vi "HelpOn.vi"(8 "Error In":errorcluster, 11 "object in":refnum<class "HelpInterface.lvclass">) -> (0 "Error Out":errorcluster, 3 "object out":refnum<class "HelpInterface.lvclass">)   [LabVIEW 2020, in "HelpInterface.lvclass"]
uses:
  HelpInterface.lvclass
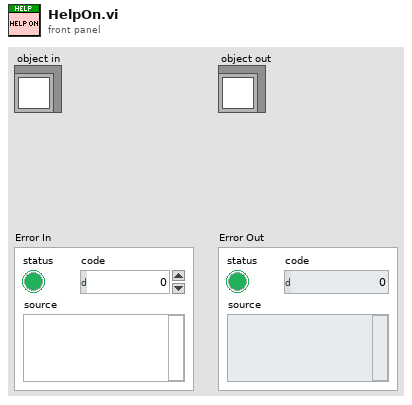
[diagram p1: front panel]
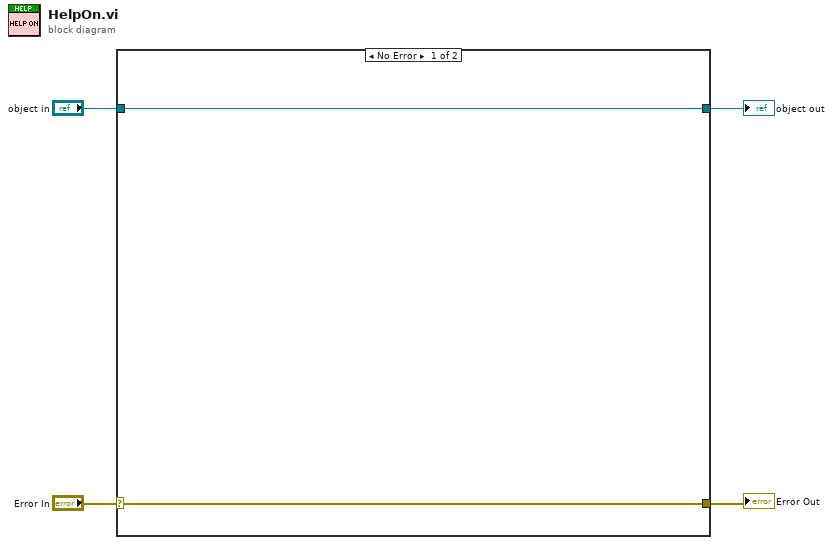
[diagram p0: block diagram]
diagram:
  n1 = case shown="No Error" "Error In" {
    selector: "Error In" -> [w5 w8]
    tunnel: [w5 w8] -> w3
    tunnel: [w6 w7] -> w1
    tunnel: "object in" -> [w6 w7]
    frame No Error {
    }
    frame Error {
    }
  }
  "Error Out" <- w3
  "object out" <- w1
